vi "test-trapezoid-profile-backwards.vi"() -> ()   [LabVIEW 2019]
uses:
  <vilib>/Rock Robotics/WPI/ThirdParty/JAS_Junk/TrajLib/TRAPEZOID_PROFILE_STATE.ctl
  <vilib>/Rock Robotics/WPI/ThirdParty/JAS_Junk/TrajLib/TRAPEZOID_PROFILE.ctl
  <vilib>/Rock Robotics/WPI/ThirdParty/JAS_Junk/TrajLib/TRAPEZOID_PROFILE_CONSTRAINT.ctl
  <vilib>/Rock Robotics/WPI/ThirdParty/JAS_Junk/TrajLib/TrapProfile_ShouldFlipAcceleration.vi
  <vilib>/Rock Robotics/WPI/ThirdParty/JAS_Junk/TrajLib/TrapProfile_Direct.vi
  <vilib>/Rock Robotics/WPI/ThirdParty/JAS_Junk/TrajLib/Trajectory_Library.lvlib
panel:
  out "TRAPEZOID_PROFILE":T1 {"Goal"."Velocity" format="%16_6e"; "Goal"."Position" format="%16_6e"; "Initial"."Velocity" format="%16_6e"; "Initial"."Position" format="%16_6e"; "Constraints"."MaxAcceleration" format="%16_6e"; "Constraints"."MaxVelocity" format="%16_6e"; "EndDecel" format="%16_6e"; "EndFullSpeed" format="%16_6e"; "EndAccel" format="%16_6e"}
  out "State":T3 {"Velocity" format="%16_6e"; "Position" format="%16_6e"}
  out "Waveform Chart":T4(graph)
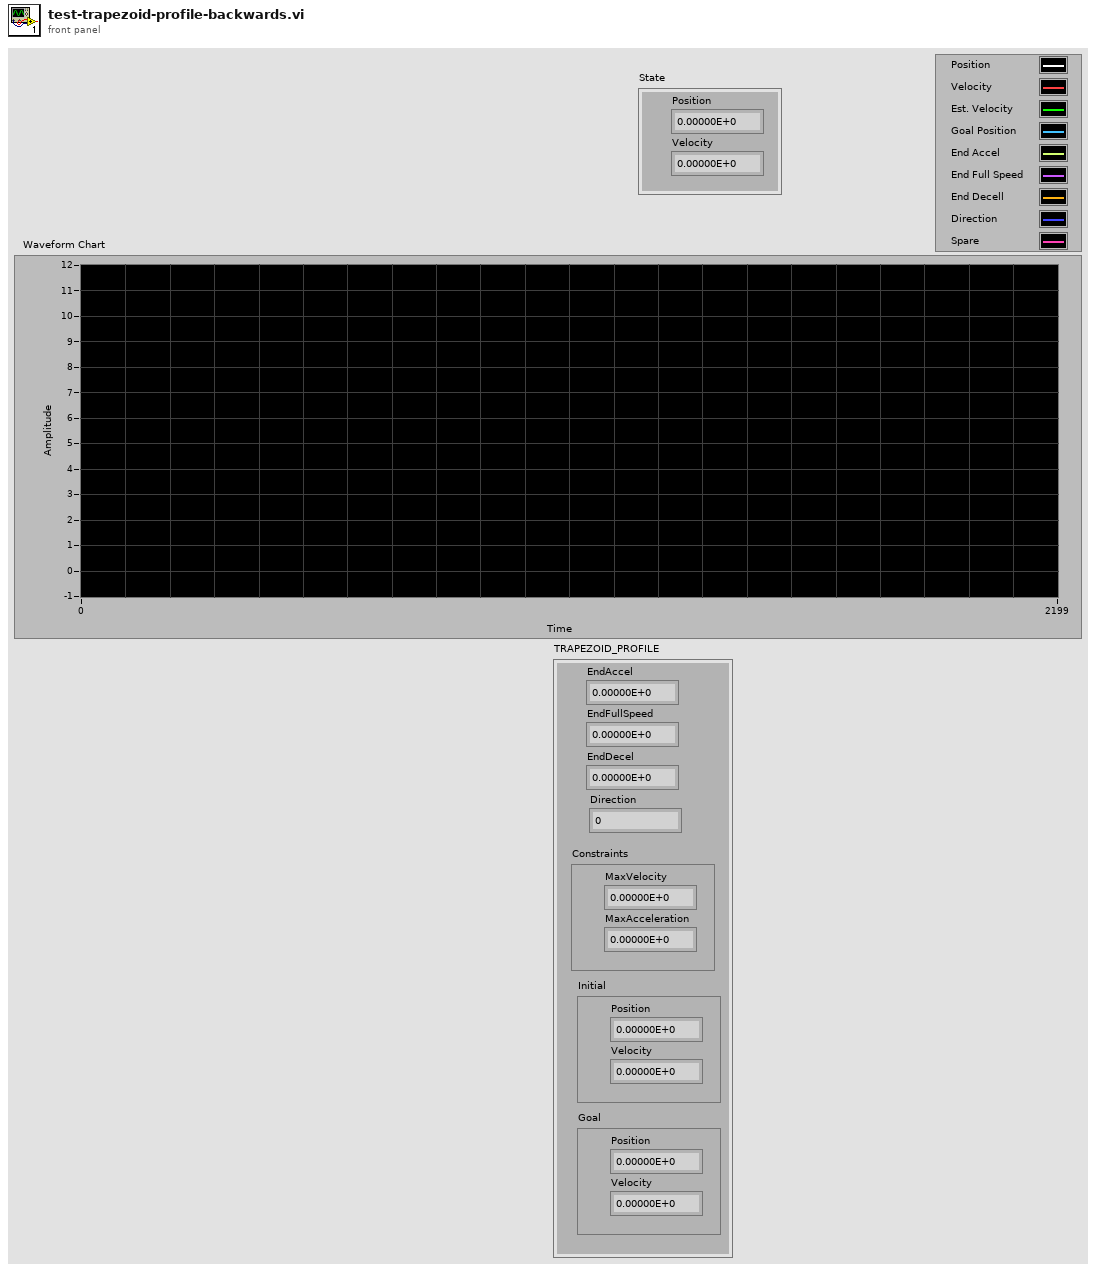
[diagram p1: front panel]
types:
  T1 = typedef "Trajectory_Library.lvlib/TRAPEZOID_PROFILE.ctl" = cluster{"EndAccel":dbl, "EndFullSpeed":dbl, "EndDecel":dbl, "Direction":i32, "Constraints":T2, "Initial":T3, "Goal":T3}
  T2 = typedef "Trajectory_Library.lvlib/TRAPEZOID_PROFILE_CONSTRAINT.ctl" = cluster{"MaxVelocity":dbl, "MaxAcceleration":dbl}
  T3 = typedef "Trajectory_Library.lvlib/TRAPEZOID_PROFILE_STATE.ctl" = cluster{"Position":dbl, "Velocity":dbl}
  T4 = cluster{"Position":dbl, "Velocity":dbl, dbl, "Position":dbl, "EndAccel":dbl, "EndFullSpeed":dbl, "EndDecel":dbl, "Direction":i32, "Position":dbl}
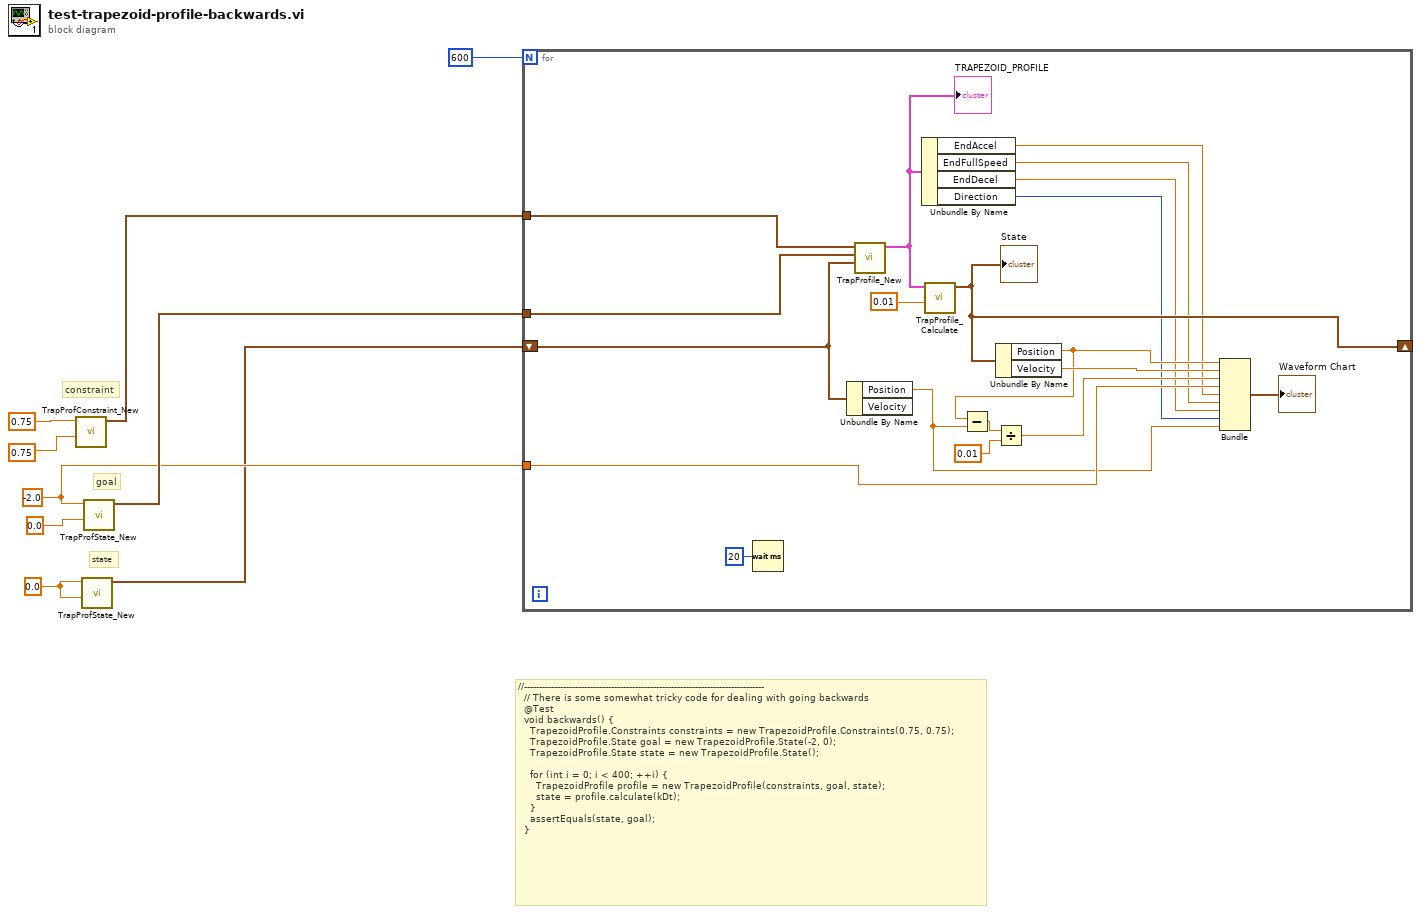
[diagram p0: block diagram]
diagram:
  w2 = 0.0 ("Position")
  w3 = -2.0 ("Position")
  # "state"
  # "//--------------------------------------------------------------------------------\n  // There is some somewhat tricky code for dealing with going backwards\n  @Test\n  void backwards() {\n    TrapezoidProfile.Constraints constraints = new TrapezoidProfile.Constraints(0.75, 0.75);\n    TrapezoidProfile.State goal = new TrapezoidProfile.State(-2, 0);\n    TrapezoidProfile.State state = new TrapezoidProfile.State();\n\n    for (int i = 0; i < 400; ++i) {\n      TrapezoidProfile profile = new TrapezoidProfile(constraints, goal, state);\n      state = profile.calculate(kDt);\n    }\n    assertEquals(state, goal);\n  }"
  # "goal"
  # "constraint"
  n1 = call <vilib>:"TrapProfConstraint_New.vi"("Max Accel"=0.75, "Max Speed (M/S)"=0.75) -> ("TRAPEZOID_PROFILE_CONSTRAINT"=w5:T2)  [unwired: 9 in]
  n2 = call <vilib>:"TrapProfState_New.vi"("Velocity"=w2, "Position"=w2) -> ("TRAPEZOID_PROFILE_STATE"=w1:T3)  [unwired: 9 in]
  n3 = call <vilib>:"TrapProfState_New.vi"("Velocity"=0.0, "Position"=w3) -> ("TRAPEZOID_PROFILE_STATE"=w4:T3)  [unwired: 9 in]
  n4 = for {
    N: 600 -> [_]
    shift-right: [w18] -> _
    shift-left: w1 -> [w23]
    tunnel: w4 -> [w25]
    tunnel: w3 -> [w17]
    tunnel: w5 -> [w10]
    n5 = Wait (ms)(milliseconds to wait=u32 20) -> ()  [unwired: 1 out]
    n6 = Unbundle By Name(w23) -> ("Position"=w11:dbl)  [unwired: 1 out]
    n7 = call <vilib>:"TrapProfile_New.vi"("Initial"=w23, "Goal"=w25, "Constraints"=w10) -> ("TRAPEZOID_PROFILE"=w16:T1)  [unwired: 8 in]
    "TRAPEZOID_PROFILE" <- w16
    n8 = Unbundle By Name(w16) -> ("EndAccel"=w15:dbl, "EndFullSpeed"=w14:dbl, "EndDecel"=w13:dbl, "Direction"=w12:i32)
    n9 = call <vilib>:"TrapProfile_Calculate.vi"("Time"=0.01, "TRAPEZOID_PROFILE"=w16) -> ("State"=w18:T3)  [unwired: 9 in]
    "State" <- w18
    n10 = Unbundle By Name(w18) -> ("Position"=w22:dbl, "Velocity"=w26:dbl)
    n11 = Subtract(x=w22, y=w11) -> (x-y=w21:dbl)
    n12 = Divide(x=w21, y=0.01) -> (x/y=w19:dbl)
    n13 = Bundle("Position"=w22, "Velocity"=w26, w19, "Position"=w17, "EndAccel"=w15, "EndFullSpeed"=w14, "EndDecel"=w13, "Direction"=w12, "Position"=w11) -> (→"Waveform Chart":T4)  [unwired: 1 in]
  }
